vi "CS POLARIS BME DG.CheckOut DG_System.vi"(8 "error IO":errorcluster, 9 "timeout in ms (-1)":i32=-1, 11 "i ref in":refnum<vi>) -> (0 "error out":errorcluster, 1 "Q timed out":bool, 2 "BME_DG_System out":refnum<class "BME_DG_System.lvclass">, 3 "i ref out":refnum<vi>)   [LabVIEW 2009, in "CS POLARIS BME DG.lvlib"]
doc: "ACHTUNG \n\nDie Funktion darf nicht nach einem Get Data to Modify Aufruf verwendet werden, sondern erst nach \nSet modified Data!!!\nDie Funktion ruft intern Get Data to Modify auf! Weitere Aufrufe von Get Data to Modify führen zu Deadlock und dürfen erst nach \"CheckIn DG_System erfolgen\"."
uses:
  CS POLARIS BME DG.lvlib
  DG Classes/BME_DG_System/BME_DG_System.lvclass
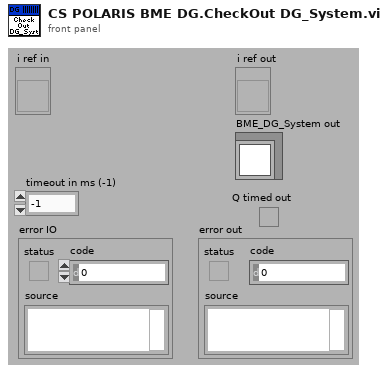
[diagram p1: front panel]
types:
  T1 = typedef "CS POLARIS BME DG.lvlib/CS POLARIS BME DG.i attribute.ctl" = cluster{"DIMLockedBy":i32, "DG_System":refnum<queue>, "UpdateTasks":refnum<queue>, "SaveEachParamChng":bool, "SaveAtShutdown":bool}
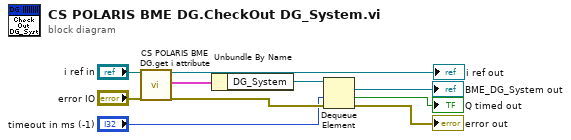
[diagram p0: block diagram]
diagram:
  n1 = call "CS POLARIS BME DG.get i attribute.vi"("i ref in"="i ref in", "error in (no error)"="error IO") -> ("i ref out"=→"i ref out":refnum<vi>, "i attribute"=w10:T1, "error out"=w8:errorcluster)  [unwired: 15 in]
  n2 = Unbundle By Name(w10) -> ("DG_System"=w1:refnum<queue>)
  n3 = Dequeue Element(queue=w1, timeout in ms (-1)="timeout in ms (-1)", error in (no error)=w8) -> (element=→"BME_DG_System out":refnum<class "BME_DG_System.lvclass">, timed out?=→"Q timed out":bool, error out=→"error out":errorcluster)  [unwired: 1 out]
